vi "Dashboard Main2.vi"() -> ()   [LabVIEW 2018]
uses:
  <vilib>/Utility/miscctls.llb/LVRowAndColumnTypeDef.ctl
  <vilib>/event_ctls.llb/eventvkey.ctl
  <vilib>/Rock Robotics/Network Tables/NT Read Numeric Array.vi
  <vilib>/Rock Robotics/WPI/Dashboard/WPI_DashboardLogging Global.vi
panel:
  in  "Camera Settings Right":T1={"Frame Rate"=30, "Compression"=30, "Size"=1, "DB Camera Config"=FALSE} {"Frame Rate" scale=1.0..30.0; "Compression" scale=100.0..-1.0; "Size" items=["640x480", "320x240", "160x120"]}
  in  "Camera Name Right":string(combo)="No Camera Selection"
  out "Camera Perf":string
  in  "Camera Settings":T1={"Frame Rate"=30, "Compression"=30, "Size"=1, "DB Camera Config"=FALSE} {"Frame Rate" scale=1.0..30.0; "Compression" scale=100.0..-1.0; "Size" items=["640x480", "320x240", "160x120"]}
  in  "TCP":refnum<k5>
  in  "Rec Mode":enum32{"Stop", "Record", "Playback"}(radio)
  out "Robot IP":string
  out "Image Message":string="Timeout in Camera Communications"
  in  "Dashboard Tab":T2(tab)
  out "Gauche":sgl(slide)
  out "Droite":sgl(slide) scale=0.0..100.0
  out "ARD":sgl(slide)
  out "ARG":sgl(slide)
  out "AVD":sgl(slide) scale=0.0..150.0
  out "AVG":sgl(slide) scale=0.0..150.0
  in  "Select Auto":string(combo)="Select Autonomous ..."
  out "NT Connection":bool
  out "Gyro":dbl(knob) scale=0.0..360.0
  out "JS1 Z":dbl(slide) scale=-1.0..1.0 scale format="%#_2e"
  out "JS1 Graph":cluster{"X":dbl, "Y":dbl}[](graph)
  out "JS1 Buttons":T3
  out "Mode":T4(ring)=enum."Auto Disabled"
  out "Right Camera Perf":cluster{"Bandwidth (Mbps)":dbl, "FPS":dbl}
  out "Camera Image Right":T5(plugin-control)
  in  "DB/String 9":string
  in  "DB/String 8":string
  in  "DB/String 7":string
  in  "DB/String 6":string
  in  "DB/String 5":string
  in  "DB/String 4":string
  in  "DB/String 3":string
  in  "DB/String 2":string
  in  "DB/String 1":string
  in  "DB/String 0":string
  in  "DB/Slider 0":dbl(slide) scale=0.0..5.0
  in  "DB/Slider 1":dbl(slide) scale=0.0..5.0
  in  "DB/Slider 2":dbl(slide) scale=0.0..5.0
  in  "DB/Slider 3":dbl(slide) scale=0.0..5.0
  out "DB/LED 3":bool
  out "DB/LED 2":bool
  out "DB/LED 1":bool
  out "DB/LED 0":bool
  in  "DB/Button 3":bool
  in  "DB/Button 2":bool
  in  "DB/Button 1":bool
  in  "DB/Button 0":bool caption="New Name"
  in  "Test Slider":dbl(slide) scale=0.0..100.0 scale format="%#_3g"
  in  "On/Off":bool caption="Solenoid"
  in  "Test Name":u16(ring) items=["Select the test to run..."]
  in  "Test Tree":string(tree)
  in  "Motor":cluster{"Value":dbl, "Enable":bool} {"Value" scale=-1.0..1.0 scale format="%#_3g"}
  out "Progress":T6 {"Test Progress" scale=0.0..100.0}
  in  "Rev/Fwd":cluster{"Forward":bool, "Reverse":bool}
  in  "Test Ring":u16(ring) items=["Monochrome", "Color"]
  out "Cmd Status":string
  in  "Execute Command":bool
  in  "Command Params":string[][](table)
  in  "Command Selection":i32(listbox)
  in  "CheckList":i32(listbox)
  out "Tree":string(tree)
  out "Camera Image":T5(plugin-control)
  in  "Camera Name":string(combo)="No Camera Selection"
  # "HW"
  # "HW"
  # "Joysticks"
  # "This tab is a great place for autonomous settings and robot-specific values.\nPlace controls and indicators inside this tab and match name to\nDashboard Variables on robot. You can also delete this comment."
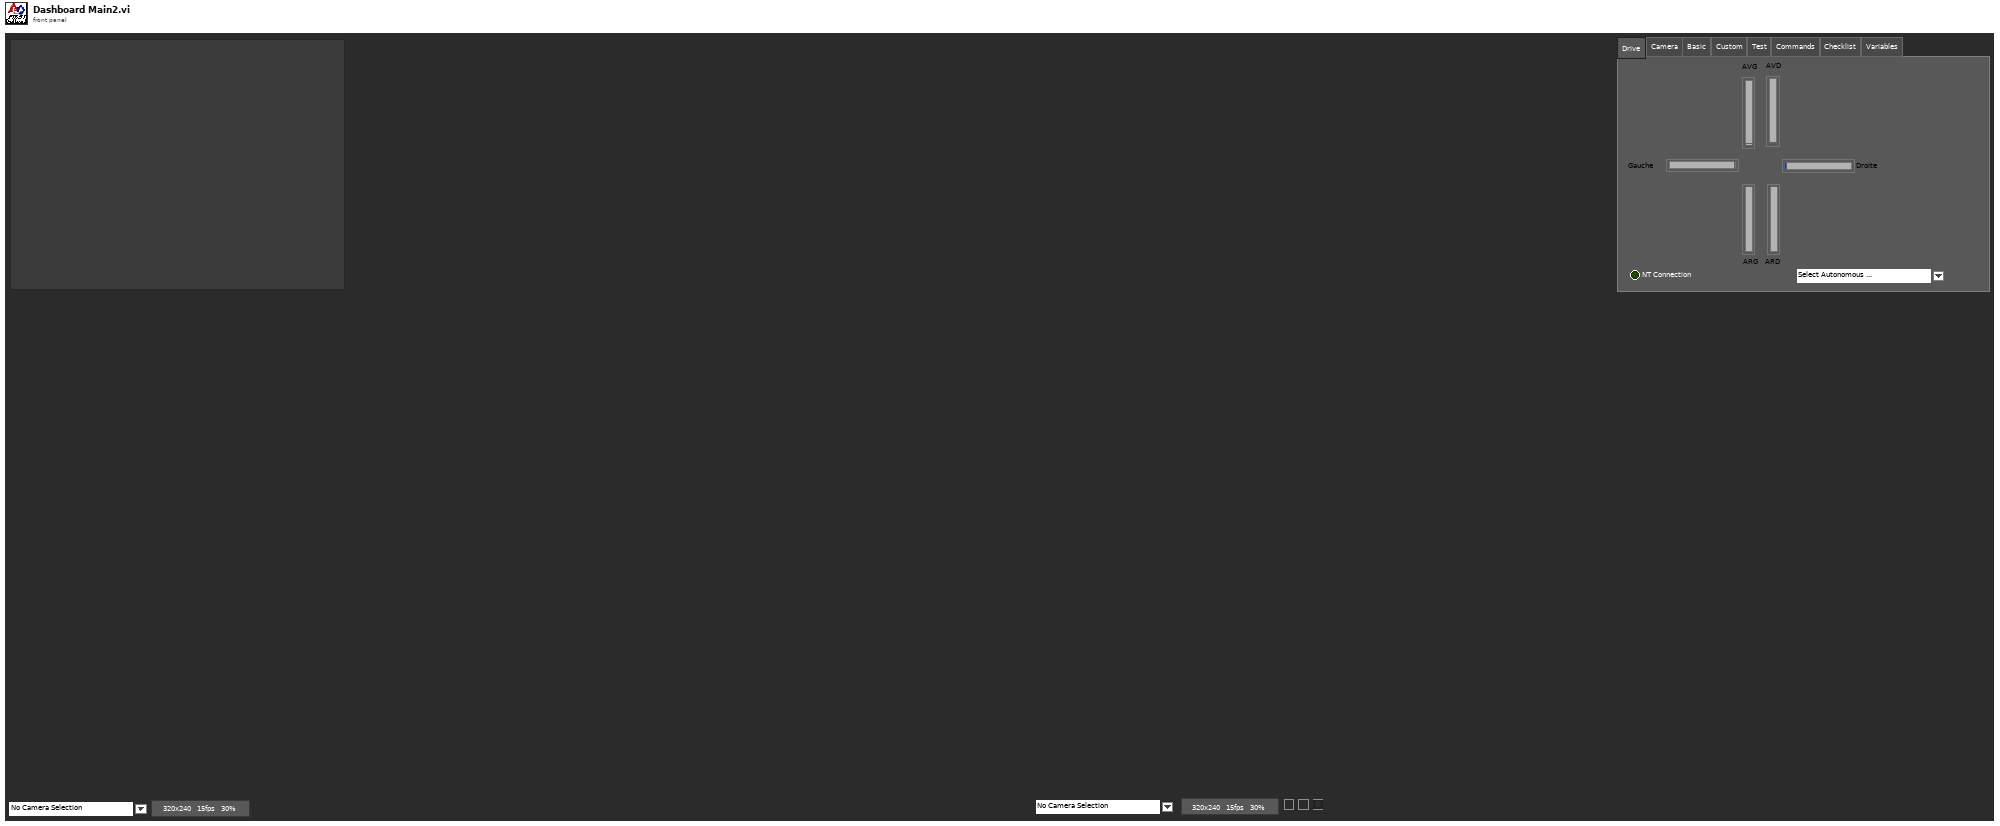
[diagram p1: front panel]
types:
  T1 = cluster{"Frame Rate":i32, "Compression":i32, "Size":u16, "DB Camera Config":bool}
  T2 = enum32{"Drive", "Camera", "Basic", "Custom", "Test", "Commands", "Checklist", "Variables"}
  T3 = cluster{bool, bool, bool, bool, bool, bool, bool, bool, bool, bool, bool, bool}
  T4 = enum8{"Tele-Op Disabled", "Tele-Op Enabled", "Auto Disabled", "Auto Enabled", "Test Disabled", "Test Enabled", "Disconnected", "No Code", "E-Stop"}
  T5 = typedef "IMAQ Image.ctl" = refnum<image>
  T6 = cluster{"Test Progress":u8, "Test Progress Text":string}
  T7 = cluster{"Save Path":path, "Interval (s)":dbl, "Keep":i32}
  T8 = typedef "Image Type" = u32
  T9 = cluster{"IDs":cluster{"RPC field ID":u16, "Unique ID":u16}, "String":string}
  T10 = cluster{"Error Strings":string, "Disable Counts":cluster{u16, u16}, "Rail Faults":cluster{u16, u16, u16}, "Robot IP":string, "DB Mode":u8, "Event Info":cluster{"Name":string, "Type":u8, "Number":u16, "Replay":u8}}
  T11 = cluster{"Storage":cluster{"Disk Free":u64, "RAM Block":u32, "RAM free":u32}, "CPU Utilization":cluster{"CPU % ISR":sgl, "CPU % Time Crit":sgl, "CPU % Timed Str":sgl, "CPU % High":sgl, "CPU % Above":sgl, "CPU % Normal":sgl, "CPU % Low":sgl}, "CAN":cluster{"% Bus Utilization":sgl, "Bus Off Cnt":u32, "TX_FIFO Full Cnt":u32, "Receive Error Cnt":u8, "Transmit Error Cnt":u8}, "HID":cluster{"HID Outputs":u32, "Rumble Low":u16, "Rumble High":u16}[]}
  T12 = cluster{"Status bits":cluster{"Test Mode":bool, "Autonomous":bool, "Enabled":bool, "Code Start":bool, "Brownout":bool, "Reserved 2":bool, "Reserved 3":bool, "E-Stop":bool}, "Code Trace":cluster{"Disabled":bool, "TeleOp":bool, "Auto":bool, "Test":bool}, "Controller Type":enum16{"unknown", "cRIO", "roboRio"}, "Code?":enum16{"unknown", "noCode", "code"}, "Battery V":dbl}
  T13 = cluster{"Control Bits":cluster{"TestMode":bool, "Autonomous":bool, "Enabled":bool, "FMS Present":bool, bool, bool, bool, "E-Stop":bool}, "Team Station ":u8, "Countdown":sgl, "Joystick Values":cluster{"Axes":dbl[], "Buttons":bool[], "POVs":i16[]}[]}
  T14 = cluster{"Axes":dbl[], "Buttons":bool[], "POVs":i16[]}[]
  T15 = cluster{"Axes":dbl[], "Buttons":bool[], "POVs":i16[]}
  T16 = cluster{"Buttons[0]":bool, "Buttons[1]":bool, "Buttons[2]":bool, "Buttons[3]":bool, "Buttons[4]":bool, "Buttons[5]":bool, "Buttons[6]":bool, "Buttons[7]":bool, "Buttons[8]":bool, "Buttons[9]":bool, "Buttons[10]":bool, "Buttons[11]":bool}
  T17 = cluster{"Camera Image":refnum<vi>, "Dashboard Tab":refnum<vi>, "Tab Button":refnum<vi>, "Rec Mode":refnum<vi>, "Test Slider":refnum<vi>, "On/Off ":refnum<vi>, "Test Ring":refnum<vi>, "Rev/Fwd":refnum<vi>, "Test Name":refnum<vi>, "Motor":refnum<vi>, "Progress":refnum<vi>, "CheckList":refnum<vi>, "Tree":refnum<vi>, "Test Tree":refnum<vi>, "Command Params":refnum<vi>, "Command Selection":refnum<vi>, "Execute Command":refnum<vi>, "Cmd Status":refnum<vi>, "Camera Settings":refnum<vi>, "Camera Name":refnum<vi>, "Camera Perf":refnum<vi>, "Camera Settings Right":refnum<vi>, "Camera Name Right":refnum<vi>, "Camera Image Right":refnum<vi>}
  T18 = cluster{"Global Rectangle":i32[], "Contours":cluster{"Contour Type":u32, "ROI Type":u32, "Points":i32[]}[]}
  T19 = cluster{"Camera Name":string, string, "Saved DB Images Info":cluster{"Save Path":path, "Interval (s)":dbl, "Keep":i32}}
  T20 = cluster{"Camera Name Right":string, string, "Saved DB Images Info":cluster{"Save Path":path, "Interval (s)":dbl, "Keep":i32}}
  T21 = cluster{"Operation":enum16{"Update", "Clear"}, "Color Box":u32}[]
  T22 = typedef "eventvkey.ctl" = enum16{"ASCII", "Enter", "Return", "Shift", "Ctrl", "Alt", "Cmd", "Opt", "Caps", "NumLock", "Clear", "Break", "Up", "Down", "Left", "Right", "Insert", "Delete", "Home", "End", "PageUp", "PageDown", "Escape", "Help", "Pause", "ScrollLock", "F1", "F2", "F3", "F4", "F5", "F6", "F7", "F8", "F9", "F10", "F11", "F12", "F13", "F14", "F15", "F16", "F17", "F18", "F19", "F20", "F21", "F22", "F23", "F24", "Play", "VolumeUp", "VolumeDown", "Mute", "Two Byte Char"}
  T23 = cluster{"Image Size":bool, "Image Type":bool, "Pixel Value":bool, "ROI Information":bool, "Zoom Factor":bool}
  T24 = cluster{"Operation":enum16{"Update", "Clear"}, "Color Box":u32}
  T25 = typedef "LVRowAndColumnTypeDef.ctl" = cluster{"Row":i32, "Column":i32}
  T26 = cluster{"Shift":bool, "Ctrl":bool, "Alt":bool, "Cmd":bool, "Opt":bool}
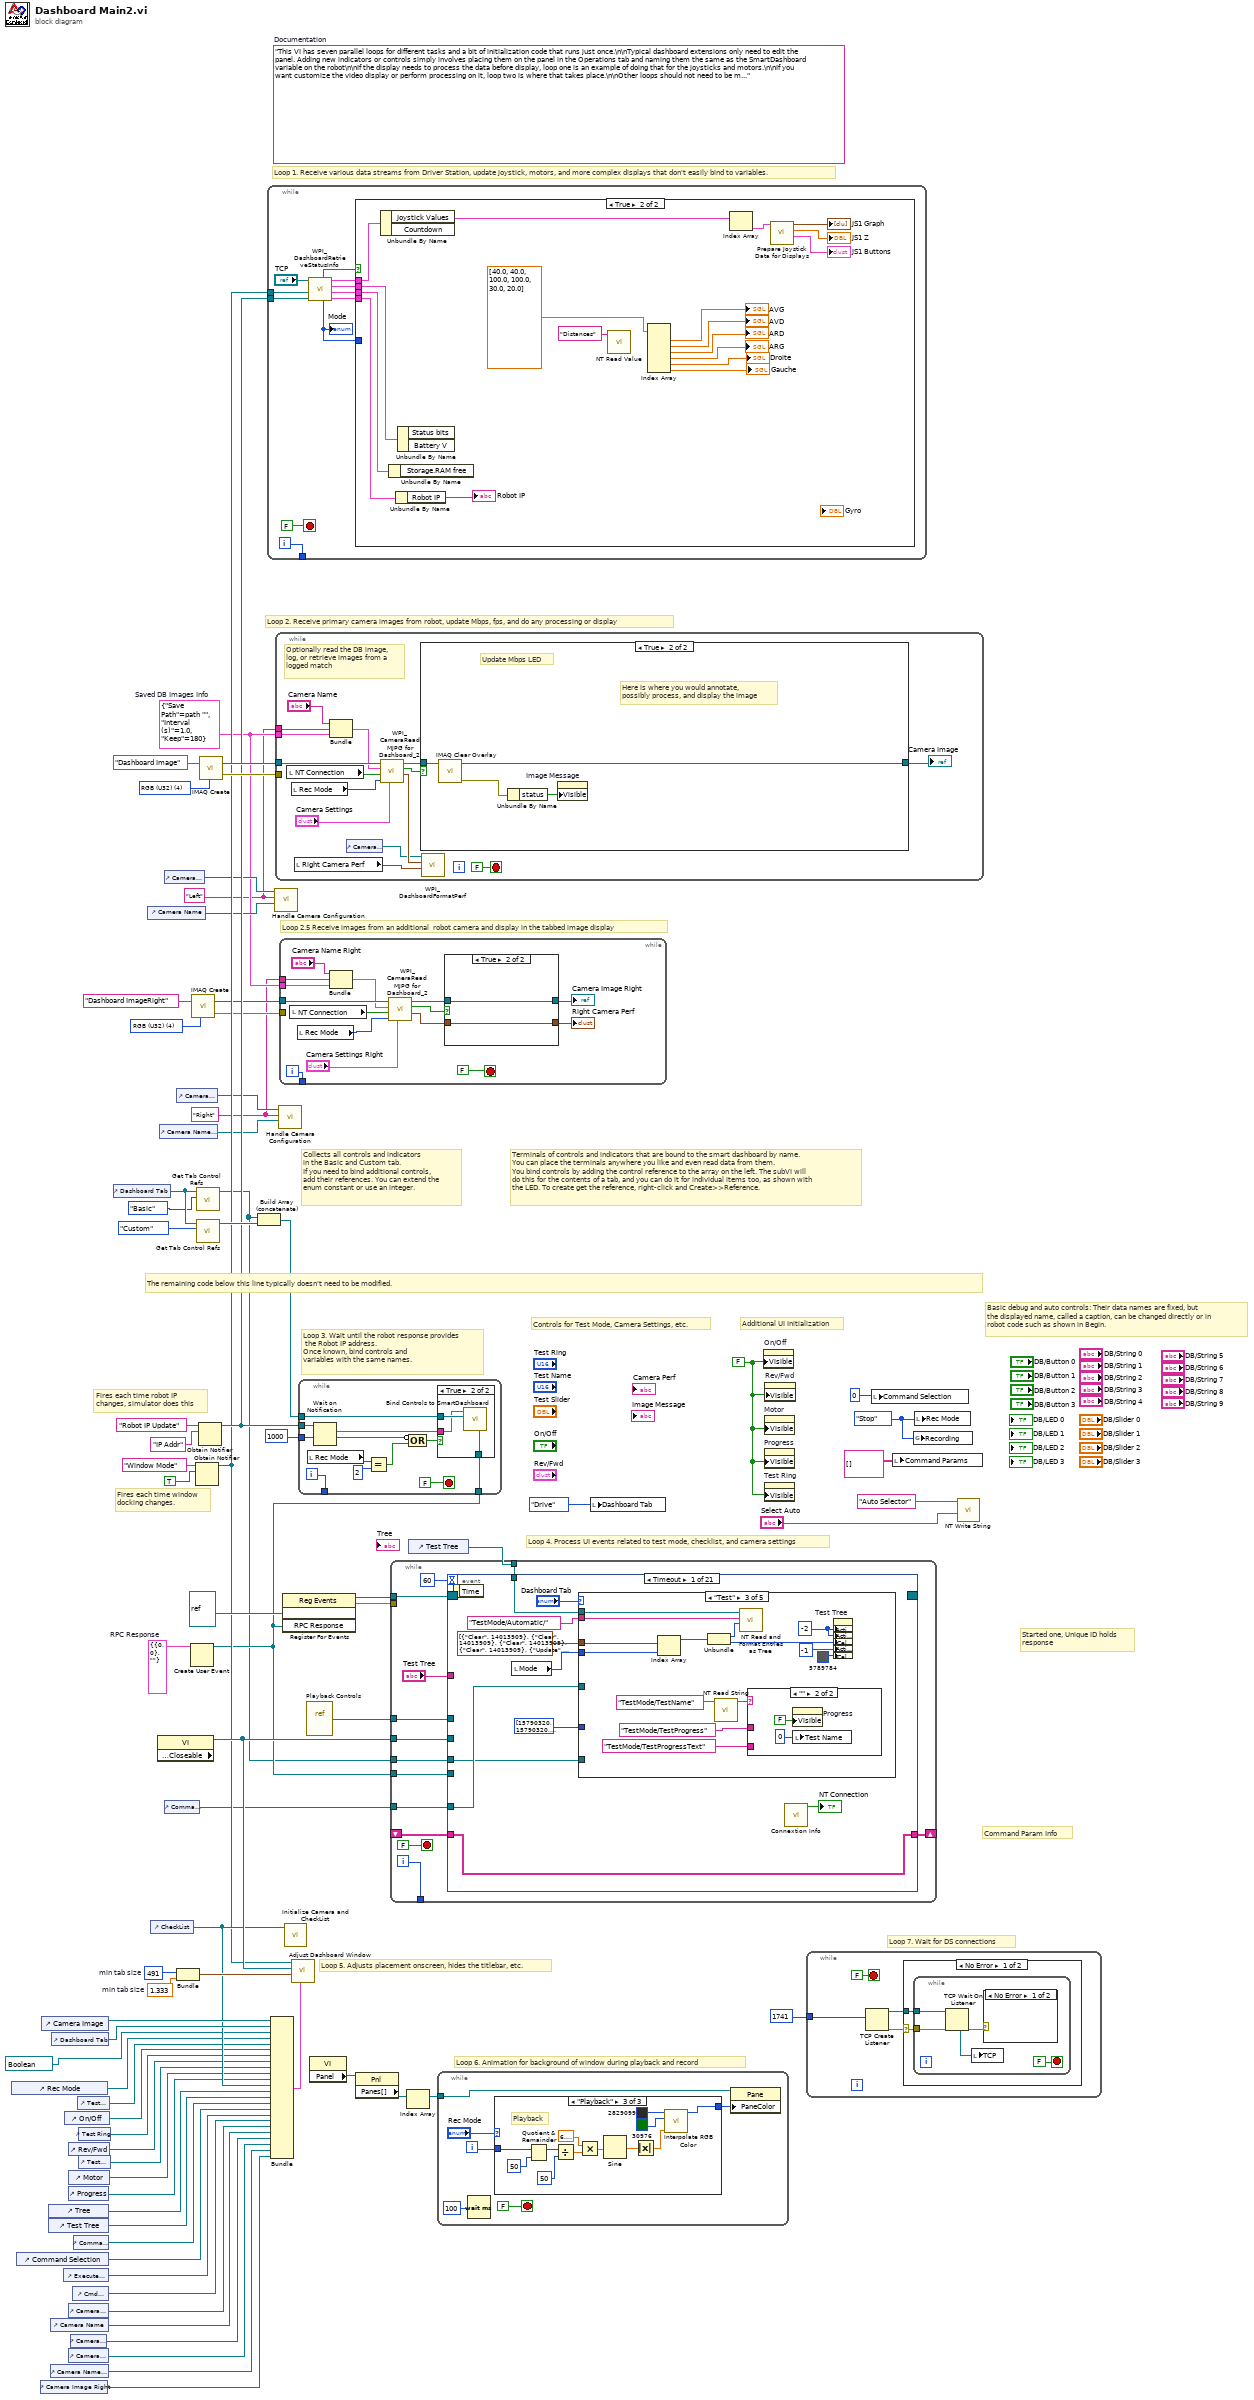
[diagram p0: block diagram]
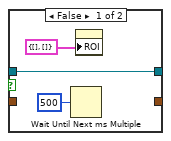
[diagram p2: hidden frame]
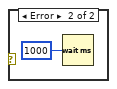
[diagram p3: hidden frame]
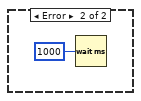
[diagram p4: hidden frame]
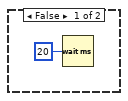
[diagram p5: hidden frame]
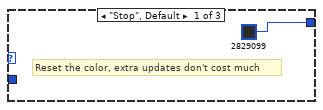
[diagram p6: hidden frame]
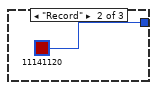
[diagram p7: hidden frame]
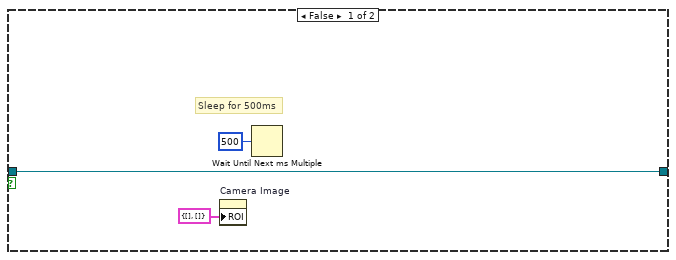
[diagram p9: hidden frame]
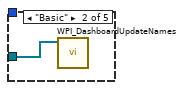
[diagram p11: hidden frame]
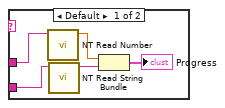
[diagram p12: hidden frame]
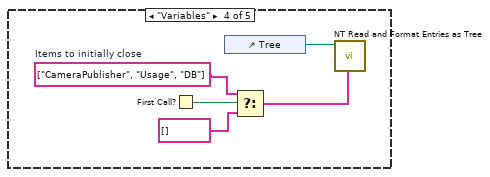
[diagram p13: hidden frame]
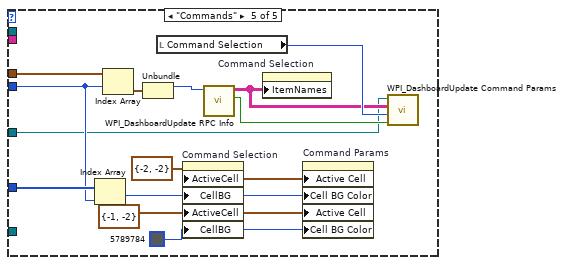
[diagram p14: hidden frame]
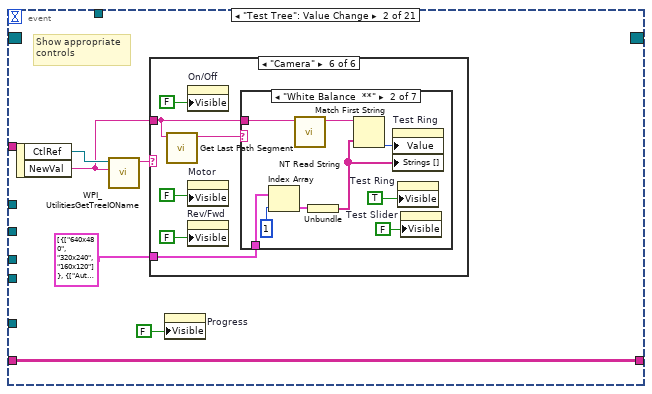
[diagram p15: hidden frame]
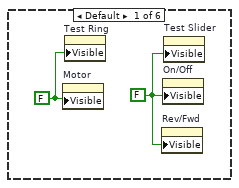
[diagram p16: hidden frame]
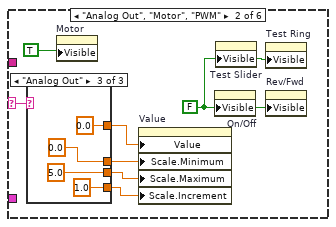
[diagram p17: hidden frame]
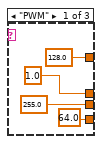
[diagram p18: hidden frame]
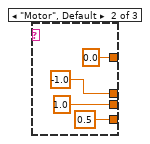
[diagram p19: hidden frame]
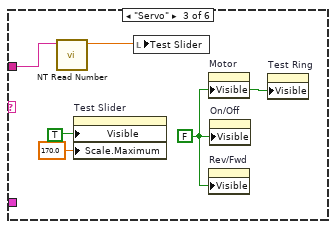
[diagram p20: hidden frame]
diagram:
  w4 = T7 {"Save Path"=path "", "Interval (s)"=1.0, "Keep"=180}  # Saved DB Images Info
  w3 = "Right"
  w2 = "Left"
  w14 = T8 4 items=["Grayscale (U8)", "Grayscale (I16)", "Grayscale (SGL)", "Complex (CSG)", "RGB (U32)", "HSL (U32)", "RGB (U64)"] ("Image Type")
  w30 = T9 {"IDs"={"RPC field ID"=0, "Unique ID"=0}, "String"=""}  # RPC Response
  w52 = 491  # min tab size
  w51 = 1.333  # min tab size
  w59 = enum32{"Stop", "Record", "Playback"}."Stop" ("Rec Mode")
  w37 = FALSE ("Visible")
  (unwired) "This VI has seven parallel loops for different tasks and a bit of initialization code that runs just once.\n\nTypical dashboard extensions only need to edit the panel. Adding new indicators or controls simply involves placing them on the panel in the Operations tab and naming them the same as the SmartDashboard variable on the robot\n\nIf the display needs to process the data before display, loop one is an example of doing that for the joysticks and motors.\n\nIf you want customize the video display or perform processing on it, loop two is where that takes place.\n\nOther loops should not need to be modified. They are pretty standard, and document the task they perform."  # Documentation
  w76 = T8 4 items=["Grayscale (U8)", "Grayscale (I16)", "Grayscale (SGL)", "Complex (CSG)", "RGB (U32)", "HSL (U32)", "RGB (U64)"] ("Image Type")
  # "Loop 2.5 Receive images from an additional  robot camera and display in the tabbed image display"
  # "Command Param Info"
  # "Started one, Unique ID holds\nresponse"
  # "Loop 7. Wait for DS connections"
  # "Basic debug and auto controls: Their data names are fixed, but\nthe displayed name, called a caption, can be changed directly or in\nrobot code such as shown in Begin."
  # "Controls for Test Mode, Camera Settings, etc."
  # "Additional UI Initialization"
  # "Loop 6. Animation for background of window during playback and record"
  # "Fires each time robot IP\nchanges, simulator does this"
  # "Fires each time window\ndocking changes."
  # "Collects all controls and indicators\nin the Basic and Custom tab.\nIf you need to bind additional controls,\nadd their references. You can extend the\nenum constant or use an integer."
  # "The remaining code below this line typically doesn't need to be modified."
  # "Loop 4. Process UI events related to test mode, checklist, and camera settings"
  # "Terminals of controls and indicators that are bound to the smart dashboard by name.\nYou can place the terminals anywhere you like and even read data from them.\nYou bind controls by adding the control reference to the array on the left. The subVI will\ndo this for the contents of a tab, and you can do it for individual items too, as shown with\nthe LED. To create get the reference, right-click and Create>>Reference."
  # "Loop 3. Wait until the robot response provides\n the Robot IP address.\nOnce known, bind controls and\nvariables with the same names."
  # "Loop 5. Adjusts placement onscreen, hides the titlebar, etc."
  # "Loop 1. Receive various data streams from Driver Station, update joystick, motors, and more complex displays that don't easily bind to variables."
  # "Loop 2. Receive primary camera images from robot, update Mbps, fps, and do any processing or display"
  n1 = control-ref of="Rec Mode"() -> (w43:refnum<vi>)
  n2 = control-ref of="Command Selection"() -> (w29:refnum<vi>)
  n3 = control-ref of="Camera Image Right"() -> (w7:refnum<vi>)
  n4 = control-ref of="Camera Image"() -> (w54:refnum<vi>)
  n5 = control-ref of="Tree"() -> (w47:refnum<vi>)
  n6 = control-ref of="Test Tree"() -> (w46:refnum<vi>)
  n7 = control-ref of="Camera Name"() -> (w20:refnum<vi>)
  n8 = control-ref of="Camera Name Right"() -> (w8:refnum<vi>)
  n9 = control-ref of="Dashboard Tab"() -> (w53:refnum<vi>)
  n10 = control-ref of="Execute Command"() -> (w31:refnum<vi>)
  n11 = control-ref of="On/Off"() -> (w41:refnum<vi>)
  n12 = control-ref of="Progress"() -> (w38:refnum<vi>)
  n13 = control-ref of="Camera Settings"() -> (w21:refnum<vi>)
  n14 = control-ref of="Camera Settings Right"() -> (w9:refnum<vi>)
  n15 = control-ref of="Rev/Fwd"() -> (w39:refnum<vi>)
  n16 = control-ref of="Motor"() -> (w44:refnum<vi>)
  n17 = control-ref of="Camera Perf"() -> (w19:refnum<vi>)
  n18 = control-ref of="Cmd Status"() -> (w25:refnum<vi>)
  n19 = control-ref of="Command Params"() -> (w32:refnum<vi>)
  n20 = control-ref of="Test Slider"() -> (w42:refnum<vi>)
  n21 = control-ref of="Test Ring"() -> (w40:refnum<vi>)
  n22 = control-ref of="Test Name"() -> (w45:refnum<vi>)
  n23 = control-ref of="Dashboard Tab"() -> (w57:refnum<vi>)
  n24 = control-ref of="Camera Name"() -> (w22:refnum<vi>)
  n25 = control-ref of="CheckList"() -> (w48:refnum<vi>)
  n26 = property class="VI" props=["Front Panel.Closeable"]() -> (reference out=w58:refnum<vi>)  [unwired: 2 in, 2 out]
  n27 = control-ref of="Camera Name Right"() -> (w10:refnum<vi>)
  n28 = control-ref of="Camera Settings"() -> (w23:refnum<vi>)
  n29 = control-ref of="Command Params"() -> (w24:refnum<vi>)
  n30 = control-ref of="Camera Settings Right"() -> (w11:refnum<vi>)
  n31 = Bundle("min tab size"=w52, "min tab size"=w51) -> (w50:cluster{"min tab size":i32, "min tab size":dbl})  [unwired: 1 in]
  n32 = Create User Event(user event datatype=w30) -> (user event=w26:refnum<user-event>)  [unwired: 1 in, 1 out]
  n33 = call "IMAQ Create"("Image Name"="Dashboard ImageRight", "Image Type"=w14) -> ("New Image"=w13:T5, "error out"=w12:errorcluster)  [unwired: 2 in, 1 out]
  n34 = Obtain Notifier(name (unnamed)="Window Mode", notification data type=TRUE) -> (notifier out=w35:refnum<notifier>)  [unwired: 2 in, 2 out]
  n35 = call <vilib>:"Get Tab Control Refs.vi"("Page Index"=T2."Basic" ("Dashboard Tab"), "TabControl in"=w57) -> ("ControlsOnPage"=w18:refnum<vi>[])  [unwired: 9 in]
  n36 = call <vilib>:"Get Tab Control Refs.vi"("Page Index"=T2."Custom" ("Dashboard Tab"), "TabControl in"=w57) -> ("ControlsOnPage"=w56:refnum<vi>[])  [unwired: 9 in]
  n37 = Obtain Notifier(name (unnamed)="Robot IP Update", notification data type="IP Addr" ("name (unnamed)")) -> (notifier out=w36:refnum<notifier>)  [unwired: 2 in, 2 out]
  n38 = call "IMAQ Create"("Image Name"="Dashboard Image", "Image Type"=w76) -> ("New Image"=w74:T5, "error out"=w73:errorcluster)  [unwired: 2 in, 1 out]
  n39 = Build Array (concatenate)(w18, w56) -> (w55:refnum<vi>[])
  n40 = while {
    tunnel: [w86] -> _
    tunnel: w36 -> [w80]
    tunnel: w35 -> [w77]
    i -> [w86]
    stop <- FALSE stop-if-true
    n41 = call <vilib>:"WPI_DashboardRetrieveStatusInfo.vi"("Binding Refnum"=w80, "Window Mode Notifier"=w77, "TCP Cnx"="TCP") -> ("Power and Errors"=w81:T10, "Robot Metrics"=w84:T11, "Status Info"=w85:T12, "Control Info"=w82:T13, "Robot Mode"=w79:T4, "Process?"=w83:bool)  [unwired: 3 in]
    "Mode" <- w79
    n42 = case shown="True" w83 {
      tunnel: w85 -> [_ w106]
      tunnel: w84 -> [_ w105]
      tunnel: w82 -> [_ w104]
      tunnel: w81 -> [_ w103]
      tunnel: w79 -> [_ _]
      frame False {
        n43 = Wait (ms)(milliseconds to wait=u32 20) -> ()  [unwired: 1 out]
      }
      frame True {
        n44 = Unbundle By Name(w104) -> ("Joystick Values"=w102:T14)  [unwired: 1 out]
        n45 = Unbundle By Name(w105) -> ()  [unwired: 1 out]
        n46 = Unbundle By Name(w103) -> ("Robot IP"=→"Robot IP":string)
        n47 = Unbundle By Name(w106) -> ()  [unwired: 2 out]
        n48 = call-poly <vilib>:"NT Read Value.vi"("Name"="Distances") -> ()  [unwired: 9 in, 2 out]
        n49 = Index Array(array=sgl[] [40.0, 40.0, 100.0, 100.0, 30.0, 20.0]) -> (element #1=→"AVG":sgl, element #2=→"AVD":sgl, element #3=→"ARD":sgl, element #4=→"ARG":sgl, element #5=→"Droite":sgl, element #6=→"Gauche":sgl)  [unwired: 6 in]
        n50 = Index Array(array=w102) -> (element=w101:T15)  [unwired: 1 in]
        n51 = call "Prepare Joystick Data for Displays.vi"("Joystick Values"=w101) -> ("Buttons"=→"JS1 Buttons":T16, "Z Axis"=→"JS1 Z":dbl, "Cartesian Data"=→"JS1 Graph":cluster{"X axis":dbl, "X axis":dbl}[])  [unwired: 8 in]
      }
    }
  }
  n52 = Bundle("Camera Image"=w54, "Dashboard Tab"=w53, "Tab Button"=refnum<vi> refnum, "Rec Mode"=w43, "Test Slider"=w42, "On/Off"=w41, "Test Ring"=w40, "Rev/Fwd"=w39, "Test Name"=w45, "Motor"=w44, "Progress"=w38, "CheckList"=w48, "Tree"=w47, "Test Tree"=w46, "Command Params"=w32, "Command Selection"=w29, "Execute Command"=w31, "Cmd Status"=w25, "Camera Settings"=w21, "Camera Name"=w20, "Camera Perf"=w19, "Camera Settings Right"=w9, "Camera Name Right"=w8, "Camera Image Right"=w7) -> (w49:T17)  [unwired: 1 in]
  n53 = call "Handle Camera Configuration.vi"("CameraNameRef"=w22, "Display Name"=w2, "ClusterRef"=w23) -> ()  [unwired: 9 in]
  n54 = while {
    tunnel: w74 -> [w120]
    tunnel: w73 -> [_]
    tunnel: w4 -> [w113]
    tunnel: w2 -> [w110]
    stop <- FALSE stop-if-true
    # "Optionally read the DB image,\nlog, or retrieve images from a\nlogged match"
    n55 = local read "NT Connection"() -> (w114:bool)
    n56 = local read "Rec Mode"() -> (w117:enum32{"Stop", "Record", "Playback"})
    n57 = local read "Right Camera Perf"() -> (w108:cluster{"Bandwidth (Mbps)":dbl, "FPS":dbl})
    n58 = Bundle("Camera Name"="Camera Name", w110, "Saved DB Images Info"=w113) -> (w112:T19)  [unwired: 1 in]
    n59 = control-ref of="Camera Perf"() -> (w107:refnum<vi>)
    n60 = call <vilib>:"WPI_CameraRead MJPG for Dashboard_2.vi"("Camera Settings"="Camera Settings", "Rec Mode"=w117, "NT Connection"=w114, "Capture Info"=w112, "Image in"=w120) -> ("perf info"=w109:cluster{"Bandwidth (Mbps)":dbl, "fps":dbl}, "Active"=w118:bool, "Image\\ out"=w119:T5)  [unwired: 4 in]
    n61 = case shown="True" w118 {
      tunnel: w119 -> [w123 w126]
      tunnel: [w123 w125] -> w115
      frame False {
        # "Sleep for 500ms"
        n62 = property on="Camera Image" class="ImageControl"("ROI"=T18 {"Global Rectangle"=[], "Contours"=[]}) -> ()  [unwired: 2 in, 2 out]
        n63 = Wait Until Next ms Multiple(millisecond multiple=u32 500) -> ()  [unwired: 1 out]
      }
      frame True {
        # "Here is where you would annotate,\npossibly process, and display the image"
        # "Update Mbps LED"
        n64 = call "IMAQ Clear Overlay"("Image"=w126) -> ("error out"=w127:errorcluster, "Image Out"=w125:T5)  [unwired: 2 in, 7 out]
        n65 = Unbundle By Name(w127) -> ("status"=w128:bool)
        n66 = property on="Image Message" class="Str"("Visible"=w128) -> ()  [unwired: 2 in, 2 out]
      }
    }
    "Camera Image" <- w115
    n67 = call <vilib>:"WPI_DashboardFormatPerf.vi"("Right Camera Perf"=w108, "Performance"=w109, "String in"=w107) -> ()  [unwired: 9 in]
  }
  n68 = call "Handle Camera Configuration.vi"("CameraNameRef"=w10, "Display Name"=w3, "ClusterRef"=w11) -> ()  [unwired: 9 in]
  n69 = while {
    tunnel: w13 -> [w143]
    tunnel: w12 -> [_]
    tunnel: [w138] -> _
    tunnel: w4 -> [w134]
    tunnel: w3 -> [w131]
    i -> [w138]
    stop <- FALSE stop-if-true
    n70 = local read "NT Connection"() -> (w135:bool)
    n71 = local read "Rec Mode"() -> (w142:enum32{"Stop", "Record", "Playback"})
    n72 = Bundle("Camera Name Right"="Camera Name Right", w131, "Saved DB Images Info"=w134) -> (w133:T20)  [unwired: 1 in]
    n73 = call <vilib>:"WPI_CameraRead MJPG for Dashboard_2.vi"("Camera Settings"="Camera Settings Right", "Rec Mode"=w142, "NT Connection"=w135, "Capture Info"=w133, "Image in"=w143) -> ("perf info"=w129:cluster{"Bandwidth (Mbps)":dbl, "fps":dbl}, "Active"=w137:bool, "Image\\ out"=w140:T5)  [unwired: 4 in]
    n74 = case shown="True" w137 {
      tunnel: w140 -> [w145 w148]
      tunnel: [w145 w148] -> w136
      tunnel: [_ w147] -> w130
      tunnel: w129 -> [_ w147]
      frame False {
        n75 = Wait Until Next ms Multiple(millisecond multiple=u32 500) -> ()  [unwired: 1 out]
        n76 = property on="Camera Image Right" class="ImageControl"("ROI"=T18 {"Global Rectangle"=[], "Contours"=[]}) -> ()  [unwired: 2 in, 2 out]
      }
      frame True {
      }
    }
    "Camera Image Right" <- w136
    "Right Camera Perf" <- w130
  }
  n77 = register-events(refnum<vi> refnum, w26) -> (reference out=w63:refnum<event-registration>, error out=w62:errorcluster)  [unwired: 2 in]
  n78 = call "Initialize Camera and CheckList.vi"("ListBox in"=w48) -> ()  [unwired: 11 in]
  n79 = call "Adjust Dashboard Window.vi"("Sizing Refnums"=w49, "Size Constraints"=w50, "VI"=w58, "WIn Mode"=w35) -> ()  [unwired: 8 in]
  n80 = while {
    tunnel: w55 -> [w160]
    tunnel: w36 -> [w158]
    tunnel: [w156] -> _
    tunnel: u32 1000 ("milliseconds to wait") -> [w155]
    tunnel: w26 -> [w149]
    i -> [w156]
    stop <- FALSE stop-if-true
    n81 = local read "Rec Mode"() -> (w151:enum32{"Stop", "Record", "Playback"})
    n82 = Wait on Notification(notifier=w158, timeout in ms (-1)=w155) -> (notification=w157:string, timed out?=w153:bool)  [unwired: 2 in, 2 out]
    n83 = Equal?(x=w151, y=u16 2 ("Rec Mode")) -> (x = y?=w152:bool)
    n84 = Compound Arithmetic op=OR(invert w153, w152) -> (w154:bool)
    n85 = case shown="True" w154 {
      tunnel: w160 -> [_ w163]
      tunnel: w157 -> [_ w162]
      tunnel: w149 -> [_ w161]
      frame False {
      }
      frame True {
        n86 = call <vilib>:"Bind Controls to SmartDashboard.vi"("RPC ref"=w161, "Bound Control Refs"=w163, "Server IP Address"=w162) -> ()  [unwired: 9 in]
      }
    }
  }
  n87 = vi-ref "Playback Controls.vi"() -> (w64:refnum<vi>)
  n88 = property class="VI"() -> ("Panel"=w66:refnum<vi>)  [unwired: 2 in, 2 out]
  n89 = property class="Pnl"(reference=w66) -> ("Panes[]"=w67:refnum<vi>[])  [unwired: 1 in, 2 out]
  n90 = Index Array(array=w67) -> (element=w65:refnum<vi>)  [unwired: 1 in]
  n91 = control-ref of="Test Tree"() -> (w68:refnum<vi>)
  n92 = while {
    tunnel: [w173] -> _
    tunnel: w68 -> [w172]
    tunnel: w64 -> [w171]
    tunnel: w63 -> [w170]
    tunnel: w62 -> [_]
    tunnel: w58 -> [w169]
    tunnel: w26 -> [w168]
    tunnel: w24 -> [w167]
    shift-right: [w166] -> _
    shift-left: _ -> [w165]
    tunnel: w18 -> [w164]
    i -> [w173]
    stop <- FALSE stop-if-true
    n93 = event shown="[0] Timeout" {
      selector: w170 -> [_ _ _ _ _ _ _ _ _ _ _ _ _ _ _ _ _ _ _ _ _]
      dyn-events: [_ _ _ _ _ _ _ _ _ _ _ _ _ _ _ _ w433 _ _ _ _] -> _
      timeout: u32 60 ("milliseconds to wait") -> [_ _ _ _ _ _ _ _ _ _ _ _ _ _ _ _ _ _ _ _ _]
      tunnel: w172 -> [w185 _ _ _ _ _ _ _ _ _ _ _ _ _ _ _ _ _ _ _ _]
      tunnel: "Test Tree" -> [_ _ _ _ _ _ _ _ _ _ _ w400 w408 w410 w414 w422 _ _ _ _ _]
      tunnel: w171 -> [_ _ _ _ _ _ _ _ _ _ _ _ _ _ _ _ w435 _ w453 _ _]
      tunnel: w169 -> [_ _ _ _ _ _ _ _ _ _ _ _ _ _ _ _ w431 _ _ _ _]
      tunnel: w168 -> [_ _ _ _ _ _ _ _ _ _ _ _ _ _ _ _ w429 _ _ _ _]
      tunnel: w167 -> [w180 _ _ _ _ _ w351 _ _ _ _ _ _ _ _ _ _ _ _ _ _]
      tunnel: [w179 w228 w330 w335 w344 w348 w349 w358 w368 w375 w387 w399 w406 w409 w413 w421 w428 w448 w450 w454 w467] -> w166
      tunnel: w165 -> [w179 w228 w330 w335 w344 w348 w349 _ _ w375 w387 w399 w406 w409 w413 w421 w428 w448 w450 w454 w467]
      tunnel: w164 -> [w177 _ _ _ _ _ _ _ _ _ _ _ _ _ _ _ _ _ _ _ _]
      event Timeout {
        n94 = event-data() -> ()  [unwired: 1 in, 1 out]
        n95 = local read "Mode"() -> (w182:T4)
        n96 = case shown="\"Test\"" "Dashboard Tab" {
          tunnel: w185 -> [_ _ w201 _ _]
          tunnel: "TestMode/Automatic/" ("Name Pattern") -> [_ _ w200 _ _]
          tunnel: T21 [{"Operation"=enum."Clear", "Color Box"=14013909}, {"Operation"=enum."Clear", "Color Box"=14013909}, {"Operation"=enum."Clear", "Color Box"=14013909}, {"Operation"=enum."Clear", "Color Box"=14013909}, {"Operation"=enum."Update", "Color Box"=14013909}, {"Operation"=enum."Update", "Color Box"=16777215}, {"Operation"=enum."Clear", "Color Box"=14013909}, {"Operation"=enum."Clear", "Color Box"=14013909}, {"Operation"=enum."Clear", "Color Box"=14013909}] -> [_ _ w193 _ w221]
          tunnel: w182 -> [_ _ w192 _ w220]
          tunnel: u32[] [15790320, 15790320, 15790320, 15790320, 16777215, 16777215, 15790320, 15790320, 15790320] -> [_ _ _ _ w226]
          tunnel: w180 -> [_ _ _ _ w214]
          tunnel: w177 -> [_ w187 _ _ _]
          frame "Custom", Default {
          }
          frame "Basic" {
            n97 = call <vilib>:"WPI_DashboardUpdateNames.vi"("Controls on Tab"=w187) -> ()  [unwired: 11 in]
          }
          frame "Test" {
            w199 = -2 ("Active Item:Row Number")
            n98 = Index Array(array=w193, index=w192) -> (element=w194:T24)
            n99 = Unbundle(w194) -> ("Operation"=w195:enum16{"Update", "Clear"}, "Color Box"=w196:u32)
            n100 = call <vilib>:"NT Read String.vi"("Name"="TestMode/TestName") -> ("String"=w190:string)  [unwired: 9 in, 1 out]
            n101 = call <vilib>:"NT Read and Format Entries as Tree.vi"("Operation"=w195, "Name Pattern"=w200, "Tree Refnum"=w201) -> ()  [unwired: 7 in, 2 out]
            n102 = case shown="\"\"" w190 {
              tunnel: "TestMode/TestProgress" ("Name") -> [w203 _]
              tunnel: "TestMode/TestProgressText" ("Name") -> [w202 _]
              frame Default {
                n103 = call <vilib>:"NT Read Number.vi"("Name"=w203) -> ("Numeric"=w204:dbl)  [unwired: 9 in, 1 out]
                n104 = call <vilib>:"NT Read String.vi"("Name"=w202) -> ("String"=w205:string)  [unwired: 9 in, 1 out]
                n105 = Bundle("Numeric"=w204, "String"=w205) -> (→"Progress":cluster{"Numeric":dbl, "String":string})  [unwired: 1 in]
              }
              frame "" {
                n106 = property on="Progress" class="Clust (strict)"("Visible"=FALSE) -> ()  [unwired: 2 in, 2 out]
                n107 = local write "Test Name"(u16 0) -> ()
              }
            }
            n108 = property on="Test Tree" class="Tree (strict)"("Active Item Row Number"=w199, "ActiveColNum"=w199, "CellBG"=w196, "Active Item Row Number"=-1 ("Active Item:Row Number"), "CellBG"=u32 5789784 ("Color Box")) -> ()  [unwired: 2 in, 2 out]
          }
          frame "Variables" {
            w211 = string[] ["CameraPublisher", "Usage", "DB"]  # Items to initially close
            n109 = First Call?() -> (First Call?: T/F=w212:bool)
            n110 = control-ref of="Tree"() -> (w213:refnum<vi>)
            n111 = Select(t=w211, s=w212, f=string[] []) -> (s? t:f=w209:string[])
            n112 = call <vilib>:"NT Read and Format Entries as Tree.vi"("Tags to  Close"=w209, "Tree Refnum"=w213) -> ()  [unwired: 8 in, 2 out]
          }
          frame "Commands" {
            w222 = u32 5789784 ("Color Box")
            w223 = T25 {"Row"=-1, "Column"=-2} ("Active Cell:Active Cell")
            w225 = T25 {"Row"=-2, "Column"=-2} ("Active Cell:Active Cell")
            n113 = Index Array(array=w226, index=w220) -> (element=w224:u32)
            n114 = Index Array(array=w221, index=w220) -> (element=w219:T24)
            n115 = Unbundle(w219) -> ("Operation"=w218:enum16{"Update", "Clear"})  [unwired: 1 out]
            n116 = local read "Command Selection"() -> (w217:i32)
            n117 = property on="Command Selection" class="MCListbox (strict)"("ActiveCell"=w225, "CellBG"=w224, "ActiveCell"=w223, "CellBG"=w222) -> ()  [unwired: 2 in, 2 out]
            n118 = call <vilib>:"WPI_DashboardUpdate RPC Info.vi"("Operation"=w218) -> ("update"=w216:bool, "commands"=w215:string[][])  [unwired: 9 in]
            n119 = property on="Command Selection" class="MCListbox (strict)"("ItemNames"=w215) -> ()  [unwired: 2 in, 2 out]
            n120 = property on="Command Params" class="Tbl (strict)"("Active Cell"=w225, "Cell BG Color"=w224, "Active Cell"=w223, "Cell BG Color"=w222) -> ()  [unwired: 2 in, 2 out]
            n121 = call <vilib>:"WPI_DashboardUpdate Command Params.vi"("Update"=w216, "NewVal"=w217, "Commands"=w215, "Param Tbl"=w214) -> ()  [unwired: 7 in, 1 out]
          }
        }
        n122 = call <vilib>:"Connextion Info.vi"() -> ("Connected"=→"NT Connection":bool)  [unwired: 10 in, 1 out]
      }
      event "Test Tree": Value Change {
        # "Show appropriate\ncontrols"
        n123 = event-data() -> ("CtlRef"=w231:refnum<vi>, "NewVal"=w229:string)  [unwired: 1 in]
        n124 = call <vilib>:"WPI_UtilitiesGetTreeIOName.vi"("NewVal"=w229, "TreeControl in"=w231) -> ("I/O Name"=w232:string)  [unwired: 9 in]
        n125 = case shown="\"Camera\"" w232 {
          selector: w232 -> [_ w239 _ w261 w270 _]
          tunnel: w229 -> [_ _ w258 w260 _ w277]
          tunnel: cluster{string[]}[] [{["640x480", "320x240", "160x120"]}, {["Auto", "Fixed indoor", "Fixed outdoor 1", "Fixed outdoor 2", "Fixed fluorescent 1", "Fixed fluorescent 2", "Hold current"]}, {["Auto", "Flicker-free 50 Hz", "Flicker-free 60 Hz", "Hold current"]}, {["None", "Prioritize frame rate", "Prioritize image quality"]}, {["Monochrome", "Color"]}] -> [_ _ _ _ _ w276]
          frame Default {
            w234 = FALSE ("Visible")
            w233 = FALSE ("Visible")
            n126 = property on="Motor" class="Clust (strict)"("Visible"=w233) -> ()  [unwired: 2 in, 2 out]
            n127 = property on="Test Ring" class="Ring (strict)"("Visible"=w233) -> ()  [unwired: 2 in, 2 out]
            n128 = property on="Rev/Fwd" class="Clust (strict)"("Visible"=w234) -> ()  [unwired: 2 in, 2 out]
            n129 = property on="On/Off" class="Bool (strict)"("Visible"=w234) -> ()  [unwired: 2 in, 2 out]
            n130 = property on="Test Slider" class="Slide (strict)"("Visible"=w234) -> ()  [unwired: 2 in, 2 out]
          }
          frame "Analog Out", "Motor", "PWM" {
            w240 = FALSE ("Visible")
            n131 = case shown="\"Analog Out\"" w239 {
              tunnel: [1.0 ("Value") -1.0 ("Value") 0.0 ("Value")] -> w238
              tunnel: [255.0 ("Value") 1.0 ("Value") 5.0 ("Value")] -> w237
              tunnel: [128.0 ("Value") 0.0 ("Value") 0.0 ("Value")] -> w236
              tunnel: [64.0 ("Value") 0.5 ("Value") 1.0 ("Value")] -> w235
              frame "PWM" {
              }
              frame "Motor", Default {
              }
              frame "Analog Out" {
              }
            }
            n132 = property on="Motor" class="Clust (strict)"("Visible"=TRUE) -> ()  [unwired: 2 in, 2 out]
            n133 = property on="Value" class="Slide (strict)"("Value"=w236, "Scale.Minimum"=w238, "Scale.Maximum"=w237, "Scale.Increment"=w235) -> ()  [unwired: 2 in, 2 out]
            n134 = property on="On/Off" class="Bool (strict)"("Visible"=w240) -> ()  [unwired: 2 in, 2 out]
            n135 = property on="Test Slider" class="Slide (strict)"("Visible"=w240) -> ()  [unwired: 2 in, 2 out]
            n136 = property on="Test Ring" class="Ring (strict)"("Visible"=w240) -> ()  [unwired: 2 in, 2 out]
            n137 = property on="Rev/Fwd" class="Clust (strict)"("Visible"=w240) -> ()  [unwired: 2 in, 2 out]
          }
          frame "Servo" {
            w256 = FALSE ("Visible")
            n138 = call <vilib>:"NT Read Number.vi"("Name"=w258) -> ("Numeric"=w257:dbl)  [unwired: 9 in, 1 out]
            n139 = property on="Test Slider" class="Slide (strict)"("Visible"=TRUE, "Scale.Maximum"=170.0 ("Scale.Range:Maximum")) -> ()  [unwired: 2 in, 2 out]
            n140 = local write "Test Slider"(w257) -> ()
            n141 = property on="Motor" class="Clust (strict)"("Visible"=w256) -> ()  [unwired: 2 in, 2 out]
            n142 = property on="Rev/Fwd" class="Clust (strict)"("Visible"=w256) -> ()  [unwired: 2 in, 2 out]
            n143 = property on="On/Off" class="Bool (strict)"("Visible"=w256) -> ()  [unwired: 2 in, 2 out]
            n144 = property on="Test Ring" class="Ring (strict)"("Visible"=w256) -> ()  [unwired: 2 in, 2 out]
          }
          frame "Relay", "Solenoid" {
            w259 = FALSE ("Visible")
            n145 = property on="Motor" class="Clust (strict)"("Visible"=w259) -> ()  [unwired: 2 in, 2 out]
            n146 = property on="Test Slider" class="Slide (strict)"("Visible"=w259) -> ()  [unwired: 2 in, 2 out]
            n147 = Search and Replace String(input string=w260, search string="/Value  **", replace string="/Direction") -> (result string=w266:string)  [unwired: 5 in, 3 out]
            n148 = property on="Test Ring" class="Ring (strict)"("Visible"=w259) -> ()  [unwired: 2 in, 2 out]
            n149 = call <vilib>:"NT Read String.vi"("Name"=w266) -> ("String"=w264:string)  [unwired: 9 in, 1 out]
            n150 = Equal?(x="Both directions", y=w264) -> (x = y?=w262:bool)
            n151 = Not(x=w262) -> (.not. x?=w263:bool)
            n152 = property on="Rev/Fwd" class="Clust (strict)"("Visible"=w262) -> ()  [unwired: 2 in, 2 out]
            n153 = property on="On/Off" class="Bool (strict)"("Visible"=w263, "Caption.Text"=w261) -> ()  [unwired: 2 in, 2 out]
          }
          frame "Compressor", "Digital Out" {
            w269 = FALSE ("Visible")
            # "Get direction and finish"
            n154 = property on="Motor" class="Clust (strict)"("Visible"=w269) -> ()  [unwired: 2 in, 2 out]
            n155 = property on="Test Slider" class="Slide (strict)"("Visible"=w269) -> ()  [unwired: 2 in, 2 out]
            n156 = property on="Test Ring" class="Ring (strict)"("Visible"=w269) -> ()  [unwired: 2 in, 2 out]
            n157 = property on="On/Off" class="Bool (strict)"("Visible"=TRUE, "Caption.Text"=w270) -> ()  [unwired: 2 in, 2 out]
            n158 = property on="Rev/Fwd" class="Clust (strict)"("Visible"=FALSE) -> ()  [unwired: 2 in, 2 out]
          }
          frame "Camera" {
            n159 = call <vilib>:"Get Last Path Segment.vi"("String in"=w277) -> ("String out"=w278:string)  [unwired: 10 in]
            n160 = property on="On/Off" class="Bool (strict)"("Visible"=FALSE) -> ()  [unwired: 2 in, 2 out]
            n161 = property on="Motor" class="Clust (strict)"("Visible"=FALSE) -> ()  [unwired: 2 in, 2 out]
            n162 = property on="Rev/Fwd" class="Clust (strict)"("Visible"=FALSE) -> ()  [unwired: 2 in, 2 out]
            n163 = case shown="\"White Balance  **\"" w278 {
              tunnel: w277 -> [w284 w293 w302 w311 w320 _ w326]
              tunnel: w276 -> [w282 w290 w299 w308 w317 _ _]
              frame "Size  **" {
                n164 = Index Array(array=w282) -> (element=w281:cluster{string[]})  [unwired: 1 in]
                n165 = call <vilib>:"NT Read String.vi"("Name"=w284) -> ("String"=w283:string)  [unwired: 9 in, 1 out]
                n166 = Unbundle(w281) -> (w279:string[])
                n167 = Match First String(2:w279, 3:w283) -> (0:w280:i32)  [unwired: 1 out]
                n168 = property on="Test Ring" class="Ring (strict)"("Value"=w280, "Strings []"=w279) -> ()  [unwired: 2 in, 2 out]
                n169 = property on="Test Ring" class="Ring (strict)"("Visible"=TRUE) -> ()  [unwired: 2 in, 2 out]
                n170 = property on="Test Slider" class="Slide (strict)"("Visible"=FALSE) -> ()  [unwired: 2 in, 2 out]
              }
              frame "White Balance  **" {
                n171 = Index Array(array=w290, index=1) -> (element=w291:cluster{string[]})
                n172 = call <vilib>:"NT Read String.vi"("Name"=w293) -> ("String"=w292:string)  [unwired: 9 in, 1 out]
                n173 = Unbundle(w291) -> (w288:string[])
                n174 = Match First String(2:w288, 3:w292) -> (0:w287:i32)  [unwired: 1 out]
                n175 = property on="Test Ring" class="Ring (strict)"("Value"=w287, "Strings []"=w288) -> ()  [unwired: 2 in, 2 out]
                n176 = property on="Test Ring" class="Ring (strict)"("Visible"=TRUE) -> ()  [unwired: 2 in, 2 out]
                n177 = property on="Test Slider" class="Slide (strict)"("Visible"=FALSE) -> ()  [unwired: 2 in, 2 out]
              }
              frame "Exposure  **" {
                n178 = Index Array(array=w299, index=2) -> (element=w300:cluster{string[]})
                n179 = call <vilib>:"NT Read String.vi"("Name"=w302) -> ("String"=w301:string)  [unwired: 9 in, 1 out]
                n180 = Unbundle(w300) -> (w296:string[])
                n181 = Match First String(2:w296, 3:w301) -> (0:w297:i32)  [unwired: 1 out]
                n182 = property on="Test Ring" class="Ring (strict)"("Value"=w297, "Strings []"=w296) -> ()  [unwired: 2 in, 2 out]
                n183 = property on="Test Ring" class="Ring (strict)"("Visible"=TRUE) -> ()  [unwired: 2 in, 2 out]
                n184 = property on="Test Slider" class="Slide (strict)"("Visible"=FALSE) -> ()  [unwired: 2 in, 2 out]
              }
              frame "Exposure Priority  **" {
                n185 = Index Array(array=w308, index=3) -> (element=w309:cluster{string[]})
                n186 = call <vilib>:"NT Read String.vi"("Name"=w311) -> ("String"=w310:string)  [unwired: 9 in, 1 out]
                n187 = Unbundle(w309) -> (w305:string[])
                n188 = Match First String(2:w305, 3:w310) -> (0:w306:i32)  [unwired: 1 out]
                n189 = property on="Test Ring" class="Ring (strict)"("Value"=w306, "Strings []"=w305) -> ()  [unwired: 2 in, 2 out]
                n190 = property on="Test Ring" class="Ring (strict)"("Visible"=TRUE) -> ()  [unwired: 2 in, 2 out]
                n191 = property on="Test Slider" class="Slide (strict)"("Visible"=FALSE) -> ()  [unwired: 2 in, 2 out]
              }
              frame "Color Enable  **" {
                n192 = Index Array(array=w317, index=4) -> (element=w318:cluster{string[]})
                n193 = call <vilib>:"NT Read String.vi"("Name"=w320) -> ("String"=w319:string)  [unwired: 9 in, 1 out]
                n194 = Unbundle(w318) -> (w314:string[])
                n195 = Match First String(2:w314, 3:w319) -> (0:w315:i32)  [unwired: 1 out]
                n196 = property on="Test Ring" class="Ring (strict)"("Value"=w315, "Strings []"=w314) -> ()  [unwired: 2 in, 2 out]
                n197 = property on="Test Ring" class="Ring (strict)"("Visible"=TRUE) -> ()  [unwired: 2 in, 2 out]
                n198 = property on="Test Slider" class="Slide (strict)"("Visible"=FALSE) -> ()  [unwired: 2 in, 2 out]
              }
              frame Default {
                n199 = property on="Test Ring" class="Ring (strict)"("Visible"=FALSE) -> ()  [unwired: 2 in, 2 out]
                n200 = property on="Test Slider" class="Slide (strict)"("Visible"=FALSE) -> ()  [unwired: 2 in, 2 out]
              }
              frame "Brightness  **", "Color Level  **", "Compression  **", "FPS  **", "Sharpness  **" {
                n201 = call <vilib>:"NT Read Number.vi"("Name"=w326) -> ("Numeric"=w325:dbl)  [unwired: 9 in, 1 out]
                n202 = local write "Test Slider"(w325) -> ()
                n203 = property on="Test Slider" class="Slide (strict)"("Visible"=TRUE, "Scale.Maximum"=100.0 ("Scale.Range:Maximum")) -> ()  [unwired: 2 in, 2 out]
                n204 = property on="Test Ring" class="Ring (strict)"("Visible"=FALSE) -> ()  [unwired: 2 in, 2 out]
              }
            }
          }
        }
        n205 = property on="Progress" class="Clust (strict)"("Visible"=FALSE) -> ()  [unwired: 2 in, 2 out]
      }
      event "Test Name": Mouse Enter {
        # "Populate the ring with the list of tests"
        n206 = event-data() -> ()  [unwired: 1 in, 1 out]
        n207 = call <vilib>:"NT Read String Array.vi"("Name"="TestMode/TestList") -> ("String Array"=w334:string[])  [unwired: 9 in, 1 out]
        n208 = Build Array (concatenate)("Select the test to run...", w334) -> (w333:string[])
        n209 = property on="Test Name" class="Ring (strict)"("Strings []"=w333) -> ()  [unwired: 2 in, 2 out]
      }
      event "Test Name": Value Change {
        w336 = FALSE ("Visible")
        # "Tell the robot the test name to run"
        n210 = event-data() -> ("NewVal"=w340:u16)  [unwired: 1 in]
        n211 = property on="Test Name" class="Ring (strict)"() -> ("Strings []"=w341:string[])  [unwired: 2 in, 2 out]
        n212 = local write "Progress"(T6 {"Test Progress"=0, "Test Progress Text"=""} ("Progress")) -> ()
        n213 = Index Array(array=w341, index=w340) -> (element=w339:string)
        n214 = call <vilib>:"NT Write String.vi"("String"=w339, "Name"="TestMode/TestName") -> ()  [unwired: 9 in, 1 out]
        n215 = property on="Progress" class="Clust (strict)"("Visible"=TRUE) -> ()  [unwired: 2 in, 2 out]
        n216 = property on="Motor" class="Clust (strict)"("Visible"=w336) -> ()  [unwired: 2 in, 2 out]
        n217 = property on="Test Slider" class="Slide (strict)"("Visible"=w336) -> ()  [unwired: 2 in, 2 out]
        n218 = property on="On/Off" class="Bool (strict)"("Visible"=w336) -> ()  [unwired: 2 in, 2 out]
        n219 = property on="Rev/Fwd" class="Clust (strict)"("Visible"=w336) -> ()  [unwired: 2 in, 2 out]
        n220 = property on="Test Ring" class="Ring (strict)"("Visible"=w336) -> ()  [unwired: 2 in, 2 out]
      }
      event "Select Auto": Mouse Enter {
        # "Populate the combo box with the list of autonomous options"
        n221 = event-data() -> ()  [unwired: 1 in, 1 out]
        n222 = call <vilib>:"NT Read String Array.vi"("Name"="Auto List") -> ("String Array"=w343:string[])  [unwired: 9 in, 1 out]
        n223 = property on="Select Auto" class="CmbBox"("Strings[]"=w343) -> ()  [unwired: 2 in, 2 out]
      }
      event "Select Auto": Value Change {
        # "User modified the Auto Selection. Write to NT variable so robot knows."
        n224 = event-data() -> ("NewVal"=w346:string)  [unwired: 1 in]
        n225 = call <vilib>:"NT Write String.vi"("String"=w346, "Name"="Auto Selector") -> ()  [unwired: 9 in, 1 out]
      }
      event "Command Selection": Value Change {
        # "Get the params and show in table"
        n226 = event-data() -> ("NewVal"=w352:i32)  [unwired: 1 in]
        n227 = property on="Command Selection" class="MCListbox (strict)"() -> ("ItemNames"=w350:string[][])  [unwired: 2 in, 2 out]
        n228 = call <vilib>:"WPI_DashboardUpdate Command Params.vi"("NewVal"=w352, "Commands"=w350, "Param Tbl"=w351) -> ()  [unwired: 8 in, 1 out]
      }
      event "Execute Command": Value Change {
        # "Started one, Unique ID holds\nresponse"
        n229 = event-data() -> ()  [unwired: 1 in, 1 out]
        n230 = property on="Command Selection" class="MCListbox (strict)"() -> ("ItemNames"=w363:string[][])  [unwired: 2 in, 2 out]
        n231 = Index Array(array=w363, index (row)="Command Selection", index (col)=0) -> (element=w361:string)
        n232 = call <vilib>:"Invoke Commands.vi"("Command Params"="Command Params", "Function Name"=w361) -> ("Params"=w357:u8, "Started"=w356:bool)  [unwired: 7 in, 1 out]
        n233 = Array Subset(array="Command Params", length (row)=w357) -> (w358:string[][])  [unwired: 3 in]
        n234 = Select(t="Executing" ("Cmd Status"), s=w356, f="" ("Cmd Status")) -> (s? t:f=→"Cmd Status":string)
      }
      event "Command Selection": Double Click {
        n235 = event-data() -> ("Row"=w371:i32)  [unwired: 1 in]
        n236 = property on="Command Selection" class="MCListbox (strict)"() -> ("ItemNames"=w374:string[][])  [unwired: 2 in, 2 out]
        n237 = local read "Command Params"() -> (w370:string[][])
        n238 = Index Array(array=w374, index (row)=w371, index (col)=0) -> (element=w372:string)
        n239 = call <vilib>:"Invoke Commands.vi"("Command Params"=w370, "Function Name"=w372) -> ("Params"=w369:u8, "Started"=w364:bool)  [unwired: 7 in, 1 out]
        n240 = Array Subset(array=w370, length (row)=w369) -> (w368:string[][])  [unwired: 3 in]
        n241 = Select(t="Executing" ("Cmd Status"), s=w364, f="" ("Cmd Status")) -> (s? t:f=w365:string)
        n242 = local write "Cmd Status"(w365) -> ()
      }
      event "CheckList": Double Click {
        # "Shift clears all"
        # "Update symbols on the listbox"
        n243 = event-data() -> ("PlatMods.Shift"=w376:bool, "Row"=w378:i32)  [unwired: 1 in]
        n244 = case shown="True" w376 {
          tunnel: w378 -> [w382 _]
          tunnel: 1 -> [w381 _]
          frame False {
            n245 = property on="CheckList" class="LstBox (strict)"() -> ("Item Symbols"=w380:i32[])  [unwired: 2 in, 2 out]
            n246 = Replace Array Subset(array=w380, new element=w381, index=w382) -> (w379:i32[])
            n247 = property on="CheckList" class="LstBox (strict)"("Item Symbols"=w379) -> ()  [unwired: 2 in, 2 out]
          }
          frame True {
            w383 = 0 ("Top Row")
            n248 = property on="CheckList" class="LstBox (strict)"() -> ("Number of Rows"=w385:u32)  [unwired: 2 in, 2 out]
            n249 = Initialize Array(0, w385) -> (w384:i32[])
            n250 = property on="CheckList" class="LstBox (strict)"("Top Row"=w383, "Value"=w383, "Item Symbols"=w384) -> ()  [unwired: 2 in, 2 out]
          }
        }
      }
      event "CheckList": Key Down {
        # "Update symbols on the listbox\nLeft and right keys check and uncheck"
        n251 = event-data() -> ("VKey"=w389:T22)  [unwired: 1 in]
        n252 = case shown="\"Left\", \"Right\"" w389 {
          selector: w389 -> [w394 _]
          tunnel: eventvkey."Left" ("VKey") -> [w392 _]
          frame "Left", "Right" {
            n253 = Equal?(x=w392, y=w394) -> (x = y?=w393:bool)
            n254 = Select(t=0, s=w393, f=1) -> (s? t:f=w395:i32)
            n255 = property on="CheckList" class="LstBox (strict)"() -> ("Item Symbols"=w398:i32[])  [unwired: 2 in, 2 out]
            n256 = Replace Array Subset(array=w398, new element=w395, index="CheckList") -> (w397:i32[])
            n257 = property on="CheckList" class="LstBox (strict)"("Item Symbols"=w397) -> ()  [unwired: 2 in, 2 out]
          }
          frame Default {
          }
        }
      }
      event "Motor.Enable": Value Change {
        # "When the test mode otor enable helper is set, update that\ntree row item's value"
        n258 = event-data() -> ("NewVal"=w404:bool)  [unwired: 1 in]
        n259 = Unbundle("Motor") -> ("Value"=w403:dbl)  [unwired: 1 out]
        n260 = Select(t=w403, s=w404, f=0.0) -> (s? t:f=w401:dbl)
        n261 = call <vilib>:"NT Write Number.vi"("Numeric"=w401, "Name"=w400) -> ()  [unwired: 9 in, 1 out]
      }
      event "Test Slider": Value Change {
        # "When the test mode slider helper is set, update that\ntree row item's value"
        n262 = event-data() -> ("NewVal"=w407:dbl)  [unwired: 1 in]
        n263 = call <vilib>:"NT Write Number.vi"("Numeric"=w407, "Name"=w408) -> ()  [unwired: 9 in, 1 out]
      }
      event "On/Off": Value Change {
        # "When the test mode on/off helper value is set, update that\ntree row item's value"
        n264 = event-data() -> ("NewVal"=w412:bool)  [unwired: 1 in]
        n265 = Boolean To (0,1)(Boolean=w412) -> (0, 1=w411:i16)
        n266 = call <vilib>:"NT Write Number.vi"("Numeric"=w411, "Name"=w410) -> ()  [unwired: 9 in, 1 out]
      }
      event "Rev/Fwd": Value Change {
        # "When the test mode helper value for relays is set, update that\ntree row item's value"
        n267 = event-data() -> ("NewVal.Forward"=w420:bool, "NewVal.Reverse"=w419:bool)  [unwired: 1 in]
        n268 = Boolean To (0,1)(Boolean=w420) -> (0, 1=w416:i16)
        n269 = Boolean To (0,1)(Boolean=w419) -> (0, 1=w418:i16)
        n270 = Negate(x=w418) -> (-x=w417:i16)
        n271 = Add(x=w416, y=w417) -> (x+y=w415:i16)
        n272 = call <vilib>:"NT Write Number.vi"("Numeric"=w415, "Name"=w414) -> ()  [unwired: 9 in, 1 out]
      }
      event "Test Ring": Value Change {
        # "When a test mode helper value is selected from the ring,\nset the tree item's variable to the string value"
        n273 = event-data() -> ("NewVal"=w424:u16)  [unwired: 1 in]
        n274 = property on="Test Ring" class="Ring (strict)"() -> ("Strings []"=w425:string[])  [unwired: 2 in, 2 out]
        n275 = Index Array(array=w425, index=w424) -> (element=w423:string)
        n276 = call <vilib>:"NT Write String.vi"("String"=w423, "Name"=w422) -> ()  [unwired: 9 in, 1 out]
      }
      event "Rec Mode": Value Change {
        # "Update globals for recording mode and path to read log from.\nClear when logging and let NetworkTables set path for vision to\nuse."
        n277 = event-data() -> ("NewVal"=w436:enum32{"Stop", "Record", "Playback"})  [unwired: 1 in]
        n278 = global write "WPI_DashboardLogging Global.vi" "Logging Filename"(path "") -> ()
        n279 = global write "WPI_DashboardLogging Global.vi" "Recording"(w436) -> ()
        n280 = case shown="\"Playback\"" w436 {
          tunnel: w435 -> [_ w438 w447]
          tunnel: [_ _ w446] -> w433
          tunnel: [_ _ w445] -> _
          tunnel: w431 -> [_ _ w443]
          tunnel: cluster{i32, i32} {-250, 170} -> [_ _ w442]
          tunnel: [_ _ T23 {"Image Size"=TRUE, "Image Type"=TRUE, "Pixel Value"=TRUE, "ROI Information"=TRUE, "Zoom Factor"=FALSE} ("Image Information Shown:All Elements")] -> w426
          tunnel: [_ _ TRUE ("Zoom Factor")] -> w427
          tunnel: w429 -> [_ _ w439]
          frame Default {
          }
          frame "Stop", "Record" {
            # "Place Window too"
            n281 = invoke class="VI" method="FP.Close"(reference=w438) -> (reference out=w437:refnum<vi>)  [unwired: 2 in, 2 out]
            n282 = invoke class="VI" method="Abort VI"(reference=w437) -> ()  [unwired: 2 in, 3 out]
          }
          frame "Playback" {
            n283 = call "Open Playback Panel.vi"("Offset"=w442, "DB VI Ref"=w443, "Playback in"=w447) -> ("Playback out"=w444:refnum<vi>)  [unwired: 8 in]
            n284 = register-events(w444, w439) -> (reference out=w446:refnum<event-registration>, error out=w445:errorcluster)  [unwired: 2 in]
          }
        }
        n285 = property on="Camera Image Right" class="ImageControl"("Image Information Shown"=w426, "Image Information Visible"=w427) -> ()  [unwired: 2 in, 2 out]
        n286 = property on="Camera Image" class="ImageControl"("Image Information Shown"=w426, "Image Information Visible"=w427) -> ()  [unwired: 2 in, 2 out]
        n287 = call <vilib>:"WPI_DashboardNT Log FieldName Cache.vi"("Operation"=enum16{"Lookup/Add", "Index", "Clear"}."Clear") -> ()  [unwired: 8 in, 3 out]
      }
      event Panel Close {
        w449 = enum32{"Stop", "Record", "Playback"}."Stop" ("Rec Mode")
        # "Playback window has been closed, abort"
        n288 = event-data() -> ()  [unwired: 1 in, 4 out]
        n289 = local write "Rec Mode"(w449) -> ()
        n290 = global write "WPI_DashboardLogging Global.vi" "Recording"(w449) -> ()
      }
      event Panel Close {
        # "Abort playback window and ourself"
        n291 = event-data() -> ()  [unwired: 1 in, 4 out]
        n292 = invoke class="VI" method="FP.Close"(reference=w453) -> (reference out=w452:refnum<vi>)  [unwired: 2 in, 2 out]
        n293 = invoke class="VI" method="Abort VI"(reference=w452) -> (error out=w451:errorcluster)  [unwired: 2 in, 2 out]
        n294 = invoke class="VI" method="Abort VI"(error in=w451) -> ()  [unwired: 2 in, 3 out]
      }
      event User Event {
        n295 = event-data() -> ("IDs"=w460:cluster{"RPC field ID":u16, "Unique ID":u16}, "String"=w459:string)  [unwired: 1 in]
        n296 = Bundle("IDs"=w460, "String"=w459) -> (w458:T9)  [unwired: 1 in]
        n297 = call <vilib>:"Retrieve RPC Response.vi"("RPC Response"=w458) -> ("Output"=w456:string[][])  [unwired: 10 in]
        n298 = Build Array (concatenate)(w454, w456) -> (w455:string[][])
        n299 = local write "Command Params"(w455) -> ()
        n300 = local write "Cmd Status"("" ("Cmd Status")) -> ()
      }
      event "Tree": Double Click {
        n301 = event-data() -> ("PlatMods"=w466:T26, "Tag"=w463:string)  [unwired: 1 in]
        n302 = Unbundle(w466) -> ("Shift"=w465:bool)  [unwired: 4 out]
        n303 = String Subset(string=w463, length (rest)=1 ("length (rest)")) -> (substring=w462:string)  [unwired: 1 in]
        n304 = Not(x=w465) -> (.not. x?=w464:bool)
        n305 = case shown="\"/\"" w462 {
          tunnel: w463 -> [_ w469]
          tunnel: w464 -> [_ w468]
          frame Default {
          }
          frame "/" {
            n306 = call <vilib>:"NT Update Persistence.vi"("Persistence"=w468, "Name"=w469) -> ()  [unwired: 9 in, 1 out]
          }
        }
      }
    }
  }
  n307 = while {
    tunnel: w65 -> [w471]
    i -> [w474]
    stop <- FALSE stop-if-true
    n308 = Wait (ms)(milliseconds to wait=u32 100) -> ()  [unwired: 1 out]
    n309 = case shown="\"Playback\"" "Rec Mode" {
      tunnel: w474 -> [_ _ w489]
      tunnel: [u32 2829099 ("Base Color") u32 11141120 ("Target Color") w478] -> w470
      frame "Stop", Default {
        # "Reset the color, extra updates don't cost much"
      }
      frame "Record" {
      }
      frame "Playback" {
        # "Playback"
        n310 = Quotient & Remainder(x=w489, y=u32 50 ("milliseconds to wait")) -> (x-y*floor(x/y)=w485:u32)  [unwired: 1 out]
        n311 = Divide(x=w485, y=u32 50 ("milliseconds to wait")) -> (x/y=w482:dbl)
        n312 = Multiply(x=6.283185307179586, y=w482) -> (x*y=w487:dbl)
        n313 = Sine(x=w487) -> (sin(x)=w486:dbl)
        n314 = Absolute Value(x=w486) -> (abs(x)=w479:dbl)
        n315 = call "Interpolate RGB Color.vi"("Proportion"=w479, "Target Color"=u32 30976, "Base Color"=u32 2829099) -> ("Result Color"=w478:u32)  [unwired: 8 in]
      }
    }
    n316 = property class="Pane"(reference=w471, "PaneColor"=w470) -> ()  [unwired: 1 in, 2 out]
  }
  n317 = local write "Dashboard Tab"(T2."Drive" ("Dashboard Tab")) -> ()
  n318 = property on="On/Off" class="Bool (strict)"("Visible"=w37) -> ()  [unwired: 2 in, 2 out]
  n319 = property on="Motor" class="Clust (strict)"("Visible"=w37) -> ()  [unwired: 2 in, 2 out]
  n320 = property on="Progress" class="Clust (strict)"("Visible"=w37) -> ()  [unwired: 2 in, 2 out]
  n321 = property on="Test Ring" class="Ring (strict)"("Visible"=w37) -> ()  [unwired: 2 in, 2 out]
  n322 = property on="Rev/Fwd" class="Clust (strict)"("Visible"=w37) -> ()  [unwired: 2 in, 2 out]
  n323 = while {
    tunnel: u16 1741 ("timeout ms (25000)") -> [w491]
    stop <- FALSE stop-if-true
    n324 = TCP Create Listener(10:w491) -> (0:w490:errorcluster, 3:w492:refnum<k5>)  [unwired: 4 in, 1 out]
    n325 = case shown="No Error" w490 {
      selector: w490 -> [w494 _]
      tunnel: w492 -> [w495 _]
      frame No Error {
        n326 = while {
          tunnel: w495 -> [w498]
          tunnel: w494 -> [w497]
          stop <- FALSE stop-if-true
          n327 = TCP Wait On Listener(8:w497, 11:w498) -> (0:w499:errorcluster, 4:w500:refnum<k5>)  [unwired: 2 in, 3 out]
          n328 = local write "TCP"(w500) -> ()
          n329 = case shown="No Error" w499 {
            frame No Error {
            }
            frame Error {
              n330 = Wait (ms)(milliseconds to wait=u32 1000) -> ()  [unwired: 1 out]
            }
          }
        }
      }
      frame Error {
        n331 = Wait (ms)(milliseconds to wait=u32 1000) -> ()  [unwired: 1 out]
      }
    }
  }
  n332 = local write "Command Selection"(u16 0 ("milliseconds to wait")) -> ()
  n333 = local write "Command Params"(string[][] [] ("Command Params")) -> ()
  n334 = global write "WPI_DashboardLogging Global.vi" "Recording"(w59) -> ()
  n335 = local write "Rec Mode"(w59) -> ()
  n336 = call <vilib>:"NT Write String.vi"("String"="Select Auto", "Name"="Auto Selector") -> ()  [unwired: 9 in, 1 out]
